vi "min_max_normalization.vi"(9 "Numeric 3":dbl, 10 "Numeric in":dbl, 11 "mean":dbl) -> (3 "Numeric out":dbl)   [LabVIEW 2020]
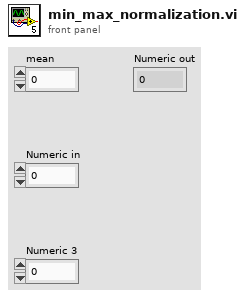
[diagram p1: front panel]
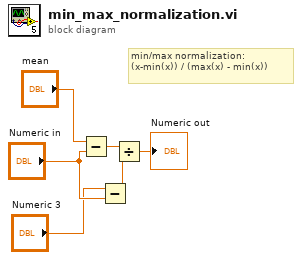
[diagram p0: block diagram]
diagram:
  # "min/max normalization: \n(x-min(x)) / (max(x) - min(x))"
  n1 = Subtract(x="mean", y="Numeric in") -> (x-y=w1:dbl)
  n2 = Subtract(x="Numeric 3", y="Numeric in") -> (x-y=w4:dbl)
  n3 = Divide(x=w1, y=w4) -> (x/y=→"Numeric out":dbl)
